vi "Read Status.vi"(8 "Error In":errorcluster, 11 "Reader In":refnum<class "Reader.lvclass">) -> (0 "Error Out":errorcluster, 2 "Status":T1, 3 "Reader Out":refnum<class "Reader.lvclass">)   [LabVIEW 2019, in "LabPack.lvlib" / "Reader.lvclass"]
doc: "Gets the latest status from the internal decoder."
uses:
  Reader.lvclass
  Controls/Status.ctl
  Reader.lvclass/Reader.ctl
  LabPack.lvlib
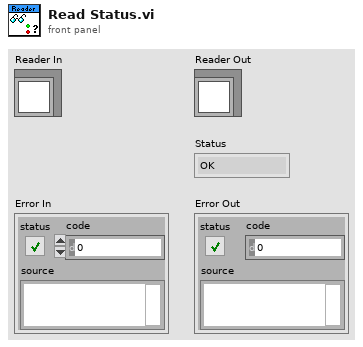
[diagram p1: front panel]
types:
  T1 = typedef "LabPack.lvlib/Status.ctl" = enum32{"OK", "Out of Memory", "Null Value", "Encoder", "Decoder"}
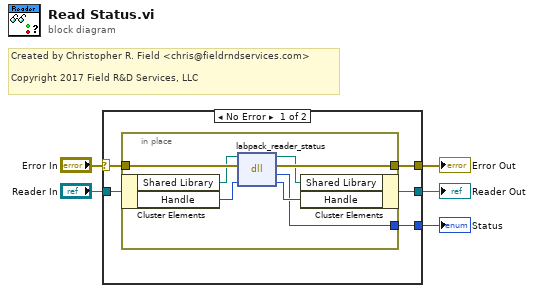
[diagram p0: block diagram]
diagram:
  # "Created by Christopher R. Field <chris@fieldrndservices.com>\n\nCopyright 2017 Field R&D Services, LLC"
  n1 = case shown="No Error" "Error In" {
    selector: "Error In" -> [w10 w19]
    tunnel: [w9 w19] -> w4
    tunnel: [w8 _] -> w3
    tunnel: "Reader In" -> [w7 w18]
    tunnel: [w6 w18] -> w1
    frame No Error {
      n2 = in-place {
        in-place-border: w10 -> [w17]
        in-place-border: [w16] -> w9
        in-place-border: [w13] -> w8
        n3 = in-place-cluster #1(w7) -> ("Shared Library"=w12:path, "Handle"=w11:u64)
        n4 = dll-call lib="D:/Users/cfield/Code/MessagePack/LabPack/LabVIEW/trunk/src/LabPack/Private/labpack-x64.dll" fn="labpack_reader_status"(path in=w12, error in=w17, "reader"=w11) -> (path out=w14:path, error out=w16:errorcluster, "return type"=w13:u32, "reader"=w15:u64)  [unwired: 1 in]
        n5 = in-place-cluster #1("Shared Library"=w14, "Handle"=w15) -> (w6:refnum<class "Reader.lvclass">)
      }
    }
    frame Error {
    }
  }
  "Error Out" <- w4
  "Status" <- w3
  "Reader Out" <- w1
